vi "FGV_leds.vi"(8 "error in":errorcluster, 10 "index":T1, 11 "action":T2=enum."read") -> (0 "error out":errorcluster, 1 "bit_state":bool, 2 "process integer":u32, 3 "state":bool[](array[boolean]), 5 "Strings []":string[](array[string]))   [LabVIEW 2018]
uses:
  controls/FGV_leds.ctl
  controls/list_of_LEDS.ctl
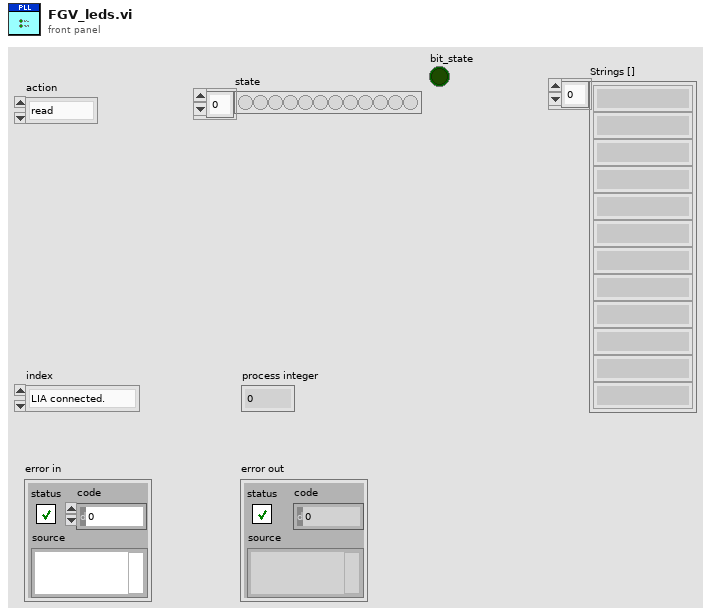
[diagram p1: front panel]
types:
  T1 = typedef "list_of_LEDS.ctl" = enum16{"LIA connected.", "Sweep in progress", "Poll in progress", "PLL enabled", "PLL locked", "Wait DAQ", "DAQ timeout", "Stop DAQ", "TDMS write"}
  T2 = typedef "FGV_leds.ctl" = enum16{"init", "read", "set bit", "clear bit", "read_bit"}
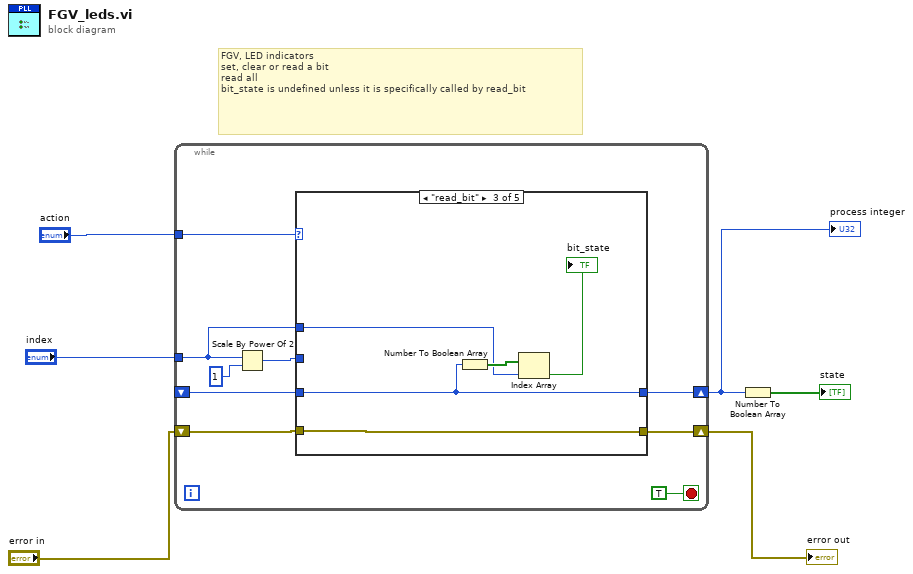
[diagram p0: block diagram]
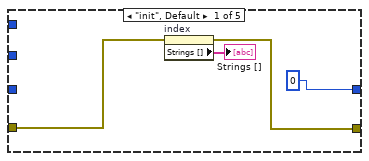
[diagram p2: hidden frame]
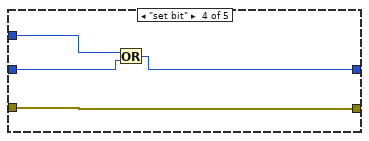
[diagram p4: hidden frame]
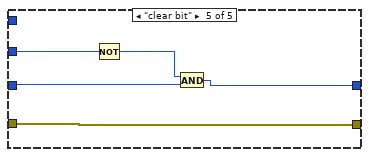
[diagram p5: hidden frame]
diagram:
  # "FGV, LED indicators\nset, clear or read a bit\nread all\nbit_state is undefined unless it is specifically called by read_bit"
  n1 = while {
    tunnel: "action" -> [w15]
    tunnel: "index" -> [w7]
    shift-right: [w14] -> w5
    shift-left: _ -> [w13]
    shift-right: [w8] -> w2
    shift-left: "error in" -> [w9]
    stop <- TRUE stop-if-true
    n2 = Scale By Power Of 2(n=w7, x=u32 1) -> (x*2^n=w12:u32)
    n3 = case shown="\"read_bit\"" w15 {
      tunnel: [u32 0 ("process") w21 w25 w28 w32] -> w14
      tunnel: w13 -> [_ w21 w25 w30 w33]
      tunnel: w12 -> [_ _ _ w29 w35]
      tunnel: w9 -> [w16 w20 w26 w27 w31]
      tunnel: [w17 w20 w26 w27 w31] -> w8
      tunnel: w7 -> [_ _ w23 _ _]
      frame "init", Default {
        n4 = property on="index" class="Enum (strict)"(error in=w16) -> (error out=w17:errorcluster, "Strings []"=→"Strings []":string[])  [unwired: 1 in, 1 out]
      }
      frame "read" {
      }
      frame "read_bit" {
        n5 = Number To Boolean Array(number=w25) -> (Boolean array=w24:bool[])
        n6 = Index Array(array=w24, index=w23) -> (element=→"bit_state":bool)
      }
      frame "set bit" {
        n7 = Or(x=w29, y=w30) -> (x .or. y?=w28:u32)
      }
      frame "clear bit" {
        n8 = Not(x=w35) -> (.not. x?=w34:u32)
        n9 = And(x=w34, y=w33) -> (x .and. y?=w32:u32)
      }
    }
  }
  "process integer" <- w5
  "error out" <- w2
  n10 = Number To Boolean Array(number=w5) -> (Boolean array=→"state":bool[])
